vi "Percent Difference.vi"(8 "Number 2":dbl, 11 "Number 1":dbl) -> (1 "Percent Difference":dbl)   [LabVIEW 2012]
doc: "This VI computes the % difference between 2 numbers according to the following formula:\nABS(x1 - x2)/Avg(x1,x2)"
panel:
  out "Average":dbl
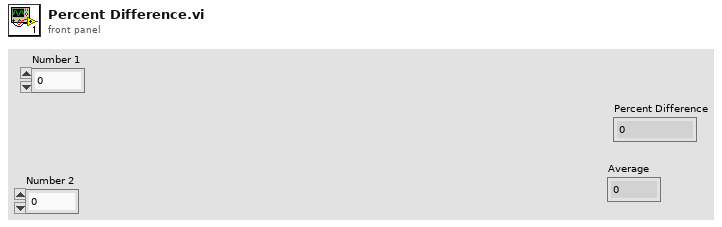
[diagram p1: front panel]
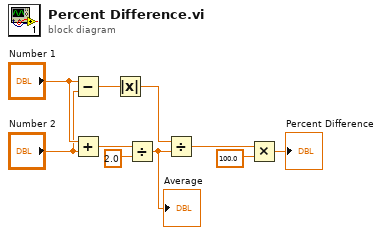
[diagram p0: block diagram]
diagram:
  n1 = Subtract(x="Number 1", y="Number 2") -> (x-y=w10:dbl)
  n2 = Add(x="Number 1", y="Number 2") -> (x+y=w7:dbl)
  n3 = Absolute Value(x=w10) -> (abs(x)=w5:dbl)
  n4 = Divide(x=w7, y=2.0) -> (x/y=w4:dbl)
  "Average" <- w4
  n5 = Divide(x=w5, y=w4) -> (x/y=w3:dbl)
  n6 = Multiply(x=w3, y=100.0) -> (x*y=→"Percent Difference":dbl)
